vi "Temp Joystick.vi"(8 "error in (no error)":errorcluster, 9 "Fiducial?":bool, 10 "Component":T1, 11 "Gantry In":refnum<k24>) -> (0 "error out":errorcluster, 2 "Error?":bool, 3 "Gantry Out":refnum<k24>)   [LabVIEW 2021, in "Component Tray.lvclass"]
uses:
  Component Tray.lvclass
  Find Component.ctl
  Controller/Camera/Machine Vision.ctl
  C:/Program Files (x86)/Aerotech/A3200/LabVIEW/2010/Bin/Aerotech.A3200.dll
  Program Files (x86)/Aerotech/A3200/LabVIEW/2010/Bin/Aerotech.A3200.dll
  Controller/Motion/A3200/A3200.lvclass
  Controller/Camera/Camera.lvclass
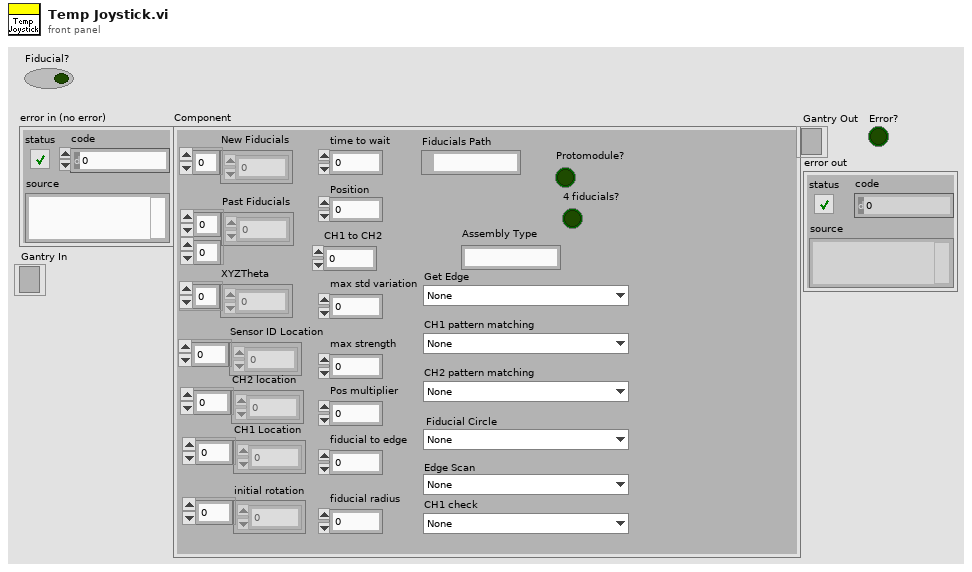
[diagram p1: front panel]
types:
  T1 = typedef "Component Tray.lvclass/Find Component.ctl" = cluster{"New Fiducials":dbl[], "Past Fiducials":dbl[][], "XYZTheta":dbl[], "Fiducials Path":path, "Position":i32, "CH1 Location":dbl[], "Sensor ID Location":dbl[], "initial rotation":dbl[], "CH2 location":dbl[], "max std variation":dbl, "max strength":dbl, "CH2 pattern matching":T2, "Fiducial Circle":T2, "Get Edge":T2, "Pos multiplier":dbl, "time to wait":u32, "fiducial to edge":dbl, "Protomodule?":bool, "Assembly Type":string, "CH1 to CH2":dbl, "Tray Number":string, "fiducial radius":dbl, "4 fiducials?":bool, "CH1 check":T2, "Edge Scan":T2, "CH1 pattern matching":T2, "Sensor Thickness":dbl}
  T2 = typedef "Camera.lvclass/Machine Vision.ctl" = enum16{"None", "Assembly Tray Circle", "Assembly Tray Fiducial", "Partial Hexaboard", "sensor edge init", "HB edge init", "sensor edge pos1", "sensor edge pos2", "HB edge pos1", "HB edge pos2", "Sensor CH1-2", "HB CH1", "HB CH2", "V3 Sensor Circle", "Hexaboard Circle", "sensor CH1 check", "HB CH1 check "}
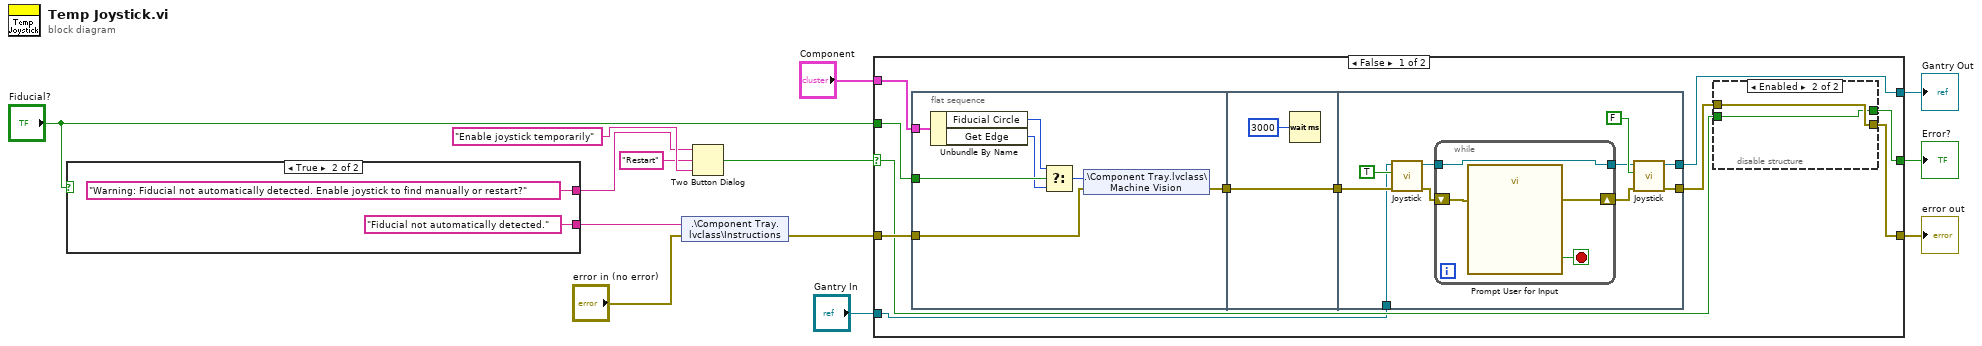
[diagram p0: block diagram]
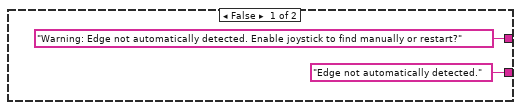
[diagram p2: hidden frame]
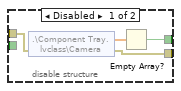
[diagram p3: hidden frame]
diagram:
  n1 = case shown="True" "Fiducial?" {
    tunnel: ["Warning: Edge not automatically detected. Enable joystick to find manually or restart?" ("message") "Warning: Fiducial not automatically detected. Enable joystick to find manually or restart?" ("message")] -> w3
    tunnel: ["Edge not automatically detected." ("Instructions") "Fiducial not automatically detected." ("Instructions")] -> w2
    frame False {
    }
    frame True {
    }
  }
  n2 = shared-variable ".\\Component Tray.lvclass\\Instructions"(w2, error in="error in (no error)") -> (error out=w13:errorcluster)
  n3 = Two Button Dialog(message=w3, 1:"Enable joystick temporarily" ("F button name (\"Cancel\")"), 2:"Restart" ("T button name (\"OK\")")) -> (T button?=w4:bool)
  n4 = case shown="False" w4 {
    selector: w4 -> [w23 w58]
    tunnel: "Gantry In" -> [w20 w60]
    tunnel: [w18 w60] -> w9
    tunnel: w13 -> [w27 w59]
    tunnel: [w26 w59] -> w8
    tunnel: "Component" -> [w28 _]
    tunnel: [w25 w58] -> w7
    tunnel: "Fiducial?" -> [w24 _]
    frame False {
      n5 = flat-sequence {
        tunnel: w28 -> [w35]
        tunnel: w27 -> [w34]
        tunnel: w24 -> [w32]
        tunnel: [w33] -> w22
        tunnel: w22 -> [w37]
        tunnel: [w37] -> w21
        tunnel: w21 -> [w47]
        tunnel: w20 -> [w45]
        tunnel: [w39] -> w19
        tunnel: [w38] -> w18
        frame #0 {
          n6 = Unbundle By Name(w35) -> ("Fiducial Circle"=w31:T2, "Get Edge"=w29:T2)
          n7 = Select(t=w31, s=w32, f=w29) -> (s? t:f=w30:T2)
          n8 = shared-variable ".\\Component Tray.lvclass\\Machine Vision"(w30, error in=w34) -> (error out=w33:errorcluster)
        }
        frame #1 {
          n9 = Wait (ms)(milliseconds to wait=u32 3000) -> ()  [unwired: 1 out]
        }
        frame #2 {
          n10 = call "Joystick.vi"("error in (no error)"=w47, "Joystick"=TRUE, "Gantry In"=w45) -> ("error out"=w43:errorcluster, "Gantry Out"=w44:refnum<k24>)  [unwired: 7 in]
          n11 = while {
            shift-right: [w49] -> w42
            shift-left: w43 -> [w50]
            tunnel: w44 -> [w51]
            tunnel: [w51] -> w40
            stop <- w48 stop-if-true
            n12 = call "Prompt User for Input"("error in (no error)"=w50) -> ("Target lined up?"=w48:bool, "error out"=w49:errorcluster)  [unwired: 16 in, 1 out]
          }
          n13 = call "Joystick.vi"("error in (no error)"=w42, "Joystick"=FALSE, "Gantry In"=w40) -> ("error out"=w39:errorcluster, "Gantry Out"=w38:refnum<k24>)  [unwired: 7 in]
        }
      }
      n14 = disable-structure shown="Enabled" {
        disable-tunnel: w19 -> [w54 w57]
        disable-tunnel: [w53 w57] -> w26
        disable-tunnel: [w52 w56] -> w25
        disable-tunnel: w23 -> [_ w56]
        frame Disabled {
          n15 = shared-variable ".\\Component Tray.lvclass\\Camera"(error in=w54) -> (w55:dbl[], error out=w53:errorcluster)
          n16 = Empty Array?(array=w55) -> (empty?=w52:bool)
        }
        frame Enabled {
        }
      }
    }
    frame True {
    }
  }
  "Gantry Out" <- w9
  "error out" <- w8
  "Error?" <- w7
